vi "Teleop.vi"(10 "Match Info":T1={"Autonomous Elapsed Seconds"=0.0, "TeleOp Elapsed Seconds"=0.0, "Disabled Elapsed Seconds"=0.0, "Visited Autonomous"=FALSE, "Visited TeleOp"=FALSE, "Visited Disabled"=FALSE, "Autonomous Settings"={"Autonomous Style"=enum."Independent", "VI Refnum"=refnum}}, 11 "Call Context":T2) -> ()   [LabVIEW 2016]
doc: "This VI is called for each TeleOp packet received from the DS where the robot is not disabled. It is often used to read from the joysticks and update I/O or to update setpoints for timed control loops. It should complete and return within 20 milliseconds or it may miss DS packets."
uses:
  <vilib>/Rock Robotics/WPI/DriverStation/WPI_DriverStationDerivedRobotMode.ctl
  <vilib>/Rock Robotics/WPI/DriverStation/WPI_DriverStationMatch Info.ctl
  <vilib>/Rock Robotics/WPI/Relay/WPI_RelayValue.ctl
  <vilib>/Rock Robotics/WPI/Solenoid/WPI_SolenoidValue.ctl
  <vilib>/Rock Robotics/WPI/Utilities/WPI_GetSetVariantRefNum.vi
  <vilib>/Rock Robotics/Network Tables/NT Write Boolean Array.vi
  <vilib>/Rock Robotics/Network Tables/NT Write Numeric Array.vi
  <vilib>/Rock Robotics/Network Tables/NT Read Boolean.vi
  <vilib>/Rock Robotics/Network Tables/NT Read Number.vi
  <vilib>/Rock Robotics/WPI/Solenoid/WPI_SolenoidSetEnum.vi
panel:
  out "Feed 2":dbl(slide) scale=-1.0..1.0
  out "Feed":dbl(slide) scale=-1.0..1.0
  out "Sample Slider 0":dbl(slide) scale=0.0..5.0
  out "Sample Boolean 1":bool
  out "Sample Boolean 0":bool
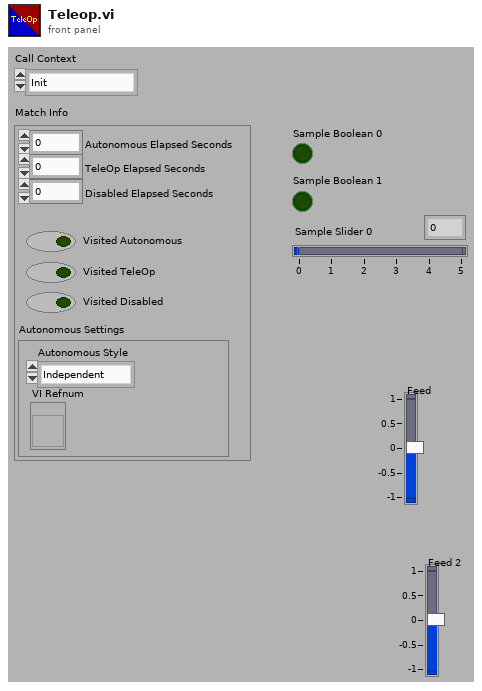
[diagram p1: front panel]
types:
  T1 = typedef "WPI_DriverStationMatch Info.ctl" = cluster{"Autonomous Elapsed Seconds":dbl, "TeleOp Elapsed Seconds":dbl, "Disabled Elapsed Seconds":dbl, "Visited Autonomous":bool, "Visited TeleOp":bool, "Visited Disabled":bool, "Autonomous Settings":cluster{"Autonomous Style":enum16{"Iterative", "Independent"}, "VI Refnum":refnum<vi>}}
  T2 = typedef "WPI_DriverStationDerivedRobotMode.ctl" = enum16{"Init", "Execute", "Stop"}
  T3 = typedef "WPI_JoystickDevRef.ctl" = cluster{"Device":T4}
  T4 = typedef "WPI_JoystickDeviceEnum.ctl" = enum16{"USB 0", "USB 1", "USB 2", "USB 3", "USB 4", "USB 5"}
  T5 = cluster{"Buttons[0]":bool, "Buttons[1]":bool, "Buttons[2]":bool, "Buttons[3]":bool, "Buttons[4]":bool, "Buttons[5]":bool, "Buttons[6]":bool, "Buttons[7]":bool, "Buttons[8]":bool, "Buttons[9]":bool, "Buttons[10]":bool}
  T6 = typedef "WPI_MotorControlDeviceRef.ctl" = cluster{"DeviceStatus":errorcluster, "Type":T7, "PWM":cluster{"PWM Channel":T8, "DeadBand":T9}, "CAN":cluster{"Device Number":u8, "SetOutput VI Ref":variant, "GetOutput VI Ref":variant, "Enable VI Ref":variant, "Disable VI Ref":variant, "Data":variant}, "Invert":bool}
  T7 = typedef "WPI_MotorControlType.ctl" = enum16{"PWM", "CAN"}
  T8 = typedef "FPGA_DIOPWMChannel.ctl" = enum8{"PWM 0", "PWM 1", "PWM 2", "PWM 3", "PWM 4", "PWM 5", "PWM 6", "PWM 7", "PWM 8", "PWM 9", "PWM MXP 0", "PWM MXP 1", "PWM MXP 2", "PWM MXP 3", "PWM MXP 4", "PWM MXP 5", "PWM MXP 6", "PWM MXP 7", "PWM MXP 8", "PWM MXP 9", "Invalid"}
  T9 = typedef "WPI_PWMDeadband.ctl" = cluster{"Name":string, "maxPositivePwm":i32, "minPositivePwm":i32, "centerPwm":i32, "maxNegativePwm":i32, "minNegativePwm":i32, "angularRange":u16}
  T10 = typedef "WPI_RelayDevRef.ctl" = cluster{"DevStatus":errorcluster, "Relay Channel":T11, "Relay Direction":T12}
  T11 = typedef "FPGA_DIORelayChannel.ctl" = enum8{"Relay 0", "Relay 1", "Relay 2", "Relay 3", "Invalid"}
  T12 = typedef "WPI_RelayDirection.ctl" = enum16{"Both directions", "Forward only", "Reverse only"}
  T13 = typedef "WPI_RobotDriveDevRef.ctl" = cluster{"DevStatus":errorcluster, "Motors[]":T6[], "Square Inputs":bool, "Max Output":dbl}
  T14 = typedef "WPI_SolenoidDevRef.ctl" = cluster{"DevStatus":errorcluster, "Pneumatics Control Module":u8, "Forward Solenoid Channel":T15, "Reverse Solenoid Channel":T15}
  T15 = typedef "WPI_SolenoidChannel.ctl" = enum8{"Solenoid 0", "Solenoid 1", "Solenoid 2", "Solenoid 3", "Solenoid 4", "Solenoid 5", "Solenoid 6", "Solenoid 7", "Invalid"}
  T16 = cluster{"Axes[0]":dbl, "Axes[1]":dbl, "Axes[2]":dbl, "Axes[3]":dbl, "Axes[4]":dbl, "Axes[5]":dbl, "Axes[6]":dbl, "Axes[7]":dbl, "Axes[8]":dbl}
  T17 = typedef "WPI_SolenoidValue.ctl" = enum16{"Off", "On", "Forward", "Reverse"}
  T18 = typedef "WPI_RelayValue.ctl" = enum16{"Off", "On", "Forward", "Reverse"}
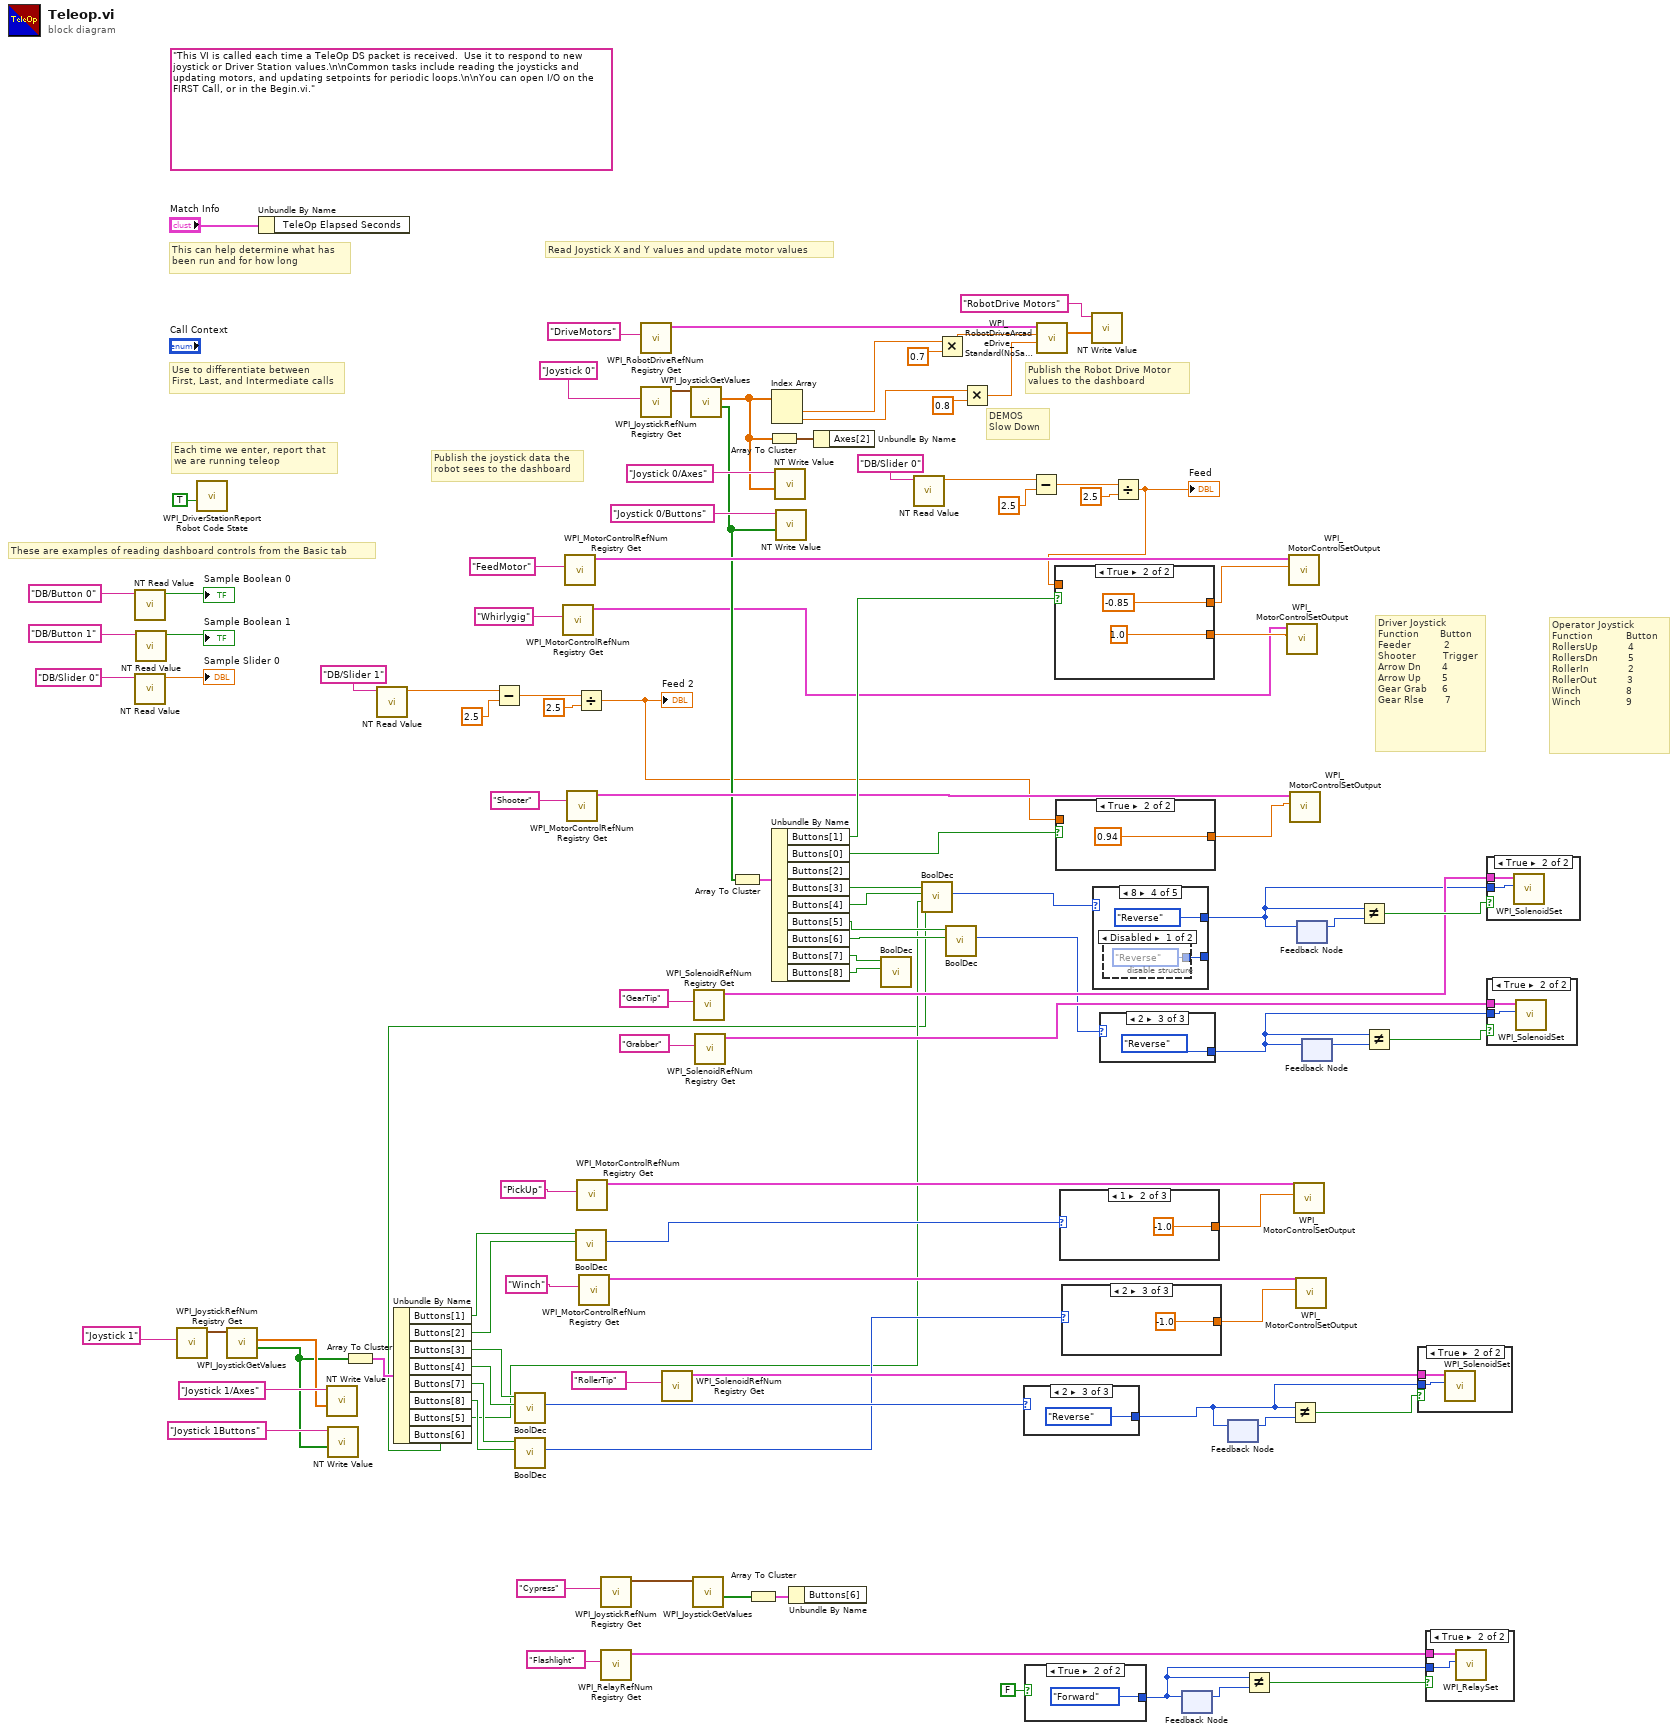
[diagram p0: block diagram]
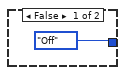
[diagram p3: hidden frame]
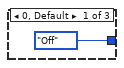
[diagram p4: hidden frame]
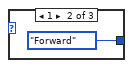
[diagram p5: hidden frame]
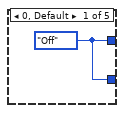
[diagram p6: hidden frame]
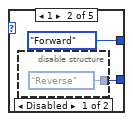
[diagram p7: hidden frame]
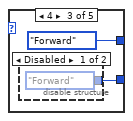
[diagram p9: hidden frame]
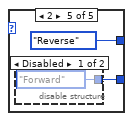
[diagram p12: hidden frame]
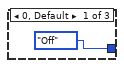
[diagram p17: hidden frame]
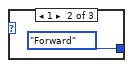
[diagram p18: hidden frame]
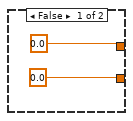
[diagram p19: hidden frame]
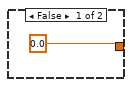
[diagram p20: hidden frame]
diagram:
  (unwired) "This VI is called each time a TeleOp DS packet is received.  Use it to respond to new joystick or Driver Station values.\n\nCommon tasks include reading the joysticks and updating motors, and updating setpoints for periodic loops.\n\nYou can open I/O on the FIRST Call, or in the Begin.vi."
  # "DEMOS\nSlow Down"
  # "Operator Joystick\nFunction           Button\nRollersUp          4\nRollersDn          5\nRollerIn             2\nRollerOut          3\nWinch               8\nWinch               9"
  # "Driver Joystick\nFunction       Button\nFeeder           2\nShooter         Trigger\nArrow Dn       4\nArrow Up       5\nGear Grab     6\nGear Rlse       7"
  # "These are examples of reading dashboard controls from the Basic tab"
  # "Publish the Robot Drive Motor\nvalues to the dashboard"
  # "Publish the joystick data the\nrobot sees to the dashboard"
  # "Each time we enter, report that\nwe are running teleop"
  # "Use to differentiate between\nFirst, Last, and Intermediate calls"
  # "This can help determine what has\nbeen run and for how long"
  # "Read Joystick X and Y values and update motor values"
  n1 = call-poly <vilib>:"NT Read Value.vi"("Name"="DB/Button 0" ("refnum name")) -> ("Boolean"=→"Sample Boolean 0":bool)  [unwired: 9 in, 1 out]
  n2 = call-poly <vilib>:"NT Read Value.vi"("Name"="DB/Slider 0" ("refnum name")) -> ("Numeric"=→"Sample Slider 0":dbl)  [unwired: 9 in, 1 out]
  n3 = call-poly <vilib>:"NT Read Value.vi"("Name"="DB/Button 1" ("refnum name")) -> ("Boolean"=→"Sample Boolean 1":bool)  [unwired: 9 in, 1 out]
  n4 = call <vilib>:"WPI_JoystickRefNum Registry Get.vi"("refnum name"="Joystick 1") -> ("JoystickDevRef"=w73:T3)  [unwired: 1 in, 9 out]
  n5 = call <vilib>:"WPI_DriverStationReport Robot Code State.vi"("TeleOp"=TRUE ("Autonomous")) -> ()  [unwired: 10 in, 1 out]
  n6 = call <vilib>:"WPI_JoystickGetValues.vi"("JoystickDevRef"=w73) -> ("Buttons"=w63:bool[], "Axes"=w69:dbl[])  [unwired: 6 in, 3 out]
  n7 = Unbundle By Name("Match Info") -> ()  [unwired: 1 out]
  n8 = call-poly <vilib>:"NT Write Value.vi"("Numeric Array"=w69, "Name"="Joystick 1/Axes") -> ()  [unwired: 9 in, 1 out]
  n9 = call-poly <vilib>:"NT Write Value.vi"("Boolean Array"=w63, "Name"="Joystick 1Buttons") -> ()  [unwired: 9 in, 1 out]
  n10 = Array To Cluster(array=w63) -> (cluster=w62:T5)
  n11 = call-poly <vilib>:"NT Read Value.vi"("Name"="DB/Slider 1") -> ("Numeric"=w37:dbl)  [unwired: 9 in, 1 out]
  n12 = Unbundle By Name(w62) -> ("Buttons[1]"=w59:bool, "Buttons[2]"=w58:bool, "Buttons[3]"=w61:bool, "Buttons[4]"=w60:bool, "Buttons[7]"=w53:bool, "Buttons[8]"=w52:bool, "Buttons[5]"=w8:bool, "Buttons[6]"=w7:bool)
  n13 = Subtract(x=w37, y=2.5) -> (x-y=w35:dbl)
  n14 = call "BoolDec.vi"("Bit0"=w61, "Bit1"=w60) -> ("Out"=w22:i8)  [unwired: 8 in]
  n15 = call "BoolDec.vi"("Bit0"=w53, "Bit1"=w52) -> ("Out"=w20:i8)  [unwired: 8 in]
  n16 = call <vilib>:"WPI_MotorControlRefNum Registry Get.vi"("refnum name"="Whirlygig") -> ("MotorControlDevRef"=w4:T6)  [unwired: 9 in, 1 out]
  n17 = call <vilib>:"WPI_MotorControlRefNum Registry Get.vi"("refnum name"="FeedMotor") -> ("MotorControlDevRef"=w76:T6)  [unwired: 9 in, 1 out]
  n18 = call <vilib>:"WPI_MotorControlRefNum Registry Get.vi"("refnum name"="Shooter") -> ("MotorControlDevRef"=w77:T6)  [unwired: 9 in, 1 out]
  n19 = Divide(x=w35, y=2.5) -> (x/y=w27:dbl)
  "Feed 2" <- w27
  n20 = call "BoolDec.vi"("Bit0"=w59, "Bit1"=w58) -> ("Out"=w21:i8)  [unwired: 8 in]
  n21 = call <vilib>:"WPI_MotorControlRefNum Registry Get.vi"("refnum name"="PickUp") -> ("MotorControlDevRef"=w86:T6)  [unwired: 9 in, 1 out]
  n22 = call <vilib>:"WPI_MotorControlRefNum Registry Get.vi"("refnum name"="Winch") -> ("MotorControlDevRef"=w81:T6)  [unwired: 9 in, 1 out]
  n23 = call <vilib>:"WPI_JoystickRefNum Registry Get.vi"("refnum name"="Cypress") -> ("JoystickDevRef"=w18:T3)  [unwired: 9 in, 1 out]
  n24 = call <vilib>:"WPI_RelayRefNum Registry Get.vi"("refnum name"="Flashlight") -> ("RelayDevRef"=w32:T10)  [unwired: 9 in, 1 out]
  n25 = call <vilib>:"WPI_RobotDriveRefNum Registry Get.vi"("refnum name"="DriveMotors") -> ("RobotDriveDevRef"=w104:T13)  [unwired: 1 in, 9 out]
  n26 = call <vilib>:"WPI_JoystickRefNum Registry Get.vi"("refnum name"="Joystick 0") -> ("JoystickDevRef"=w102:T3)  [unwired: 1 in, 9 out]
  n27 = call <vilib>:"WPI_SolenoidRefNum Registry Get.vi"("refnum name"="RollerTip") -> ("SolenoidDevRef"=w64:T14)  [unwired: 9 in, 1 out]
  n28 = call <vilib>:"WPI_JoystickGetValues.vi"("JoystickDevRef"=w102) -> ("Buttons"=w68:bool[], "Axes"=w88:dbl[])  [unwired: 6 in, 3 out]
  n29 = call <vilib>:"WPI_JoystickGetValues.vi"("JoystickDevRef"=w18) -> ("Buttons"=w17:bool[])  [unwired: 6 in, 4 out]
  n30 = call <vilib>:"WPI_SolenoidRefNum Registry Get.vi"("refnum name"="GearTip") -> ("SolenoidDevRef"=w25:T14)  [unwired: 9 in, 1 out]
  n31 = call <vilib>:"WPI_SolenoidRefNum Registry Get.vi"("refnum name"="Grabber") -> ("SolenoidDevRef"=w24:T14)  [unwired: 9 in, 1 out]
  n32 = Array To Cluster(array=w68) -> (cluster=w89:T5)
  n33 = Array To Cluster(array=w17) -> (cluster=w16:T5)
  n34 = Array To Cluster(array=w88) -> (cluster=w87:T16)
  n35 = Index Array(array=w88) -> (element #1=w46:dbl, element #2=w2:dbl)  [unwired: 2 in]
  n36 = Unbundle By Name(w89) -> ("Buttons[1]"=w78:bool, "Buttons[0]"=w79:bool, "Buttons[3]"=w9:bool, "Buttons[4]"=w26:bool, "Buttons[5]"=w15:bool, "Buttons[6]"=w14:bool, "Buttons[7]"=w84:bool, "Buttons[8]"=w83:bool)  [unwired: 1 out]
  n37 = call-poly <vilib>:"NT Write Value.vi"("Numeric Array"=w88, "Name"="Joystick 0/Axes") -> ()  [unwired: 9 in, 1 out]
  n38 = call-poly <vilib>:"NT Write Value.vi"("Boolean Array"=w68, "Name"="Joystick 0/Buttons") -> ()  [unwired: 9 in, 1 out]
  n39 = Unbundle By Name(w16) -> ()  [unwired: 1 out]
  n40 = Unbundle By Name(w87) -> ()  [unwired: 1 out]
  n41 = call "BoolDec.vi"("Bit0"=w84, "Bit1"=w83) -> ()  [unwired: 8 in, 1 out]
  n42 = call-poly <vilib>:"NT Read Value.vi"("Name"="DB/Slider 0") -> ("Numeric"=w43:dbl)  [unwired: 9 in, 1 out]
  n43 = call "BoolDec.vi"("Bit0"=w9, "Bit1"=w26, "Bit2"=w8, "Bit3"=w7) -> ("Out"=w13:i8)  [unwired: 6 in]
  n44 = Multiply(x=w46, y=0.7) -> (x*y=w10:dbl)
  n45 = call "BoolDec.vi"("Bit0"=w15, "Bit1"=w14) -> ("Out"=w23:i8)  [unwired: 8 in]
  n46 = Multiply(x=w2, y=0.8) -> (x*y=w1:dbl)
  n47 = case shown="2" w22 {
    tunnel: [WPI_SolenoidValue."Off" ("Value") WPI_SolenoidValue."Forward" ("Value") WPI_SolenoidValue."Reverse" ("Value")] -> w49
    frame 0, Default {
    }
    frame 1 {
    }
    frame 2 {
    }
  }
  n48 = case shown="True" FALSE {
    tunnel: [WPI_RelayValue."Off" ("RelayValue") WPI_RelayValue."Forward" ("RelayValue")] -> w28
    frame False {
    }
    frame True {
    }
  }
  n49 = Subtract(x=w43, y=2.5) -> (x-y=w41:dbl)
  n50 = call <vilib>:"WPI_RobotDriveArcadeDrive_Standard(NoSaturation).vi"("Y axis value"=w1, "X axis value"=w10, "RobotDriveDevRef"=w104) -> ("Motor Values"=w92:dbl[])  [unwired: 1 in, 7 out]
  n51 = case shown="True" w79 {
    tunnel: [0.0 ("Output") 0.94] -> w47
    tunnel: w27 -> [_ _]
    frame False {
    }
    frame True {
    }
  }
  n52 = case shown="1" w21 {
    tunnel: [0.0 ("Output") -1.0 1.0] -> w85
    frame 0, Default {
    }
    frame 1 {
    }
    frame 2 {
    }
  }
  n53 = case shown="2" w20 {
    tunnel: [0.0 ("Output") 1.0 -1.0] -> w82
    frame 0, Default {
    }
    frame 1 {
    }
    frame 2 {
    }
  }
  n54 = call-poly <vilib>:"NT Write Value.vi"("Numeric Array"=w92, "Name"="RobotDrive Motors") -> ()  [unwired: 9 in, 1 out]
  n55 = case shown="8" w13 {
    tunnel: [w120 WPI_SolenoidValue."Forward" ("Value") WPI_SolenoidValue."Forward" ("Value") WPI_SolenoidValue."Reverse" ("Value") WPI_SolenoidValue."Reverse" ("Value")] -> w12
    tunnel: [w120 w121 w124 w127 w130] -> _
    frame 0, Default {
      w120 = WPI_SolenoidValue."Off" ("Value")
    }
    frame 1 {
      n56 = disable-structure shown="Disabled" {
        disable-tunnel: [WPI_SolenoidValue."Reverse" ("Value") _] -> w121
        frame Disabled {
        }
        frame Enabled {
        }
      }
    }
    frame 4 {
      n57 = disable-structure shown="Disabled" {
        disable-tunnel: [WPI_SolenoidValue."Forward" ("Value") _] -> w124
        frame Disabled {
        }
        frame Enabled {
        }
      }
    }
    frame 8 {
      n58 = disable-structure shown="Disabled" {
        disable-tunnel: [WPI_SolenoidValue."Reverse" ("Value") _] -> w127
        frame Disabled {
        }
        frame Enabled {
        }
      }
    }
    frame 2 {
      n59 = disable-structure shown="Disabled" {
        disable-tunnel: [WPI_SolenoidValue."Forward" ("Value") _] -> w130
        frame Disabled {
        }
        frame Enabled {
        }
      }
    }
  }
  n60 = case shown="2" w23 {
    tunnel: [WPI_SolenoidValue."Off" ("Value") WPI_SolenoidValue."Forward" ("Value") WPI_SolenoidValue."Reverse" ("Value")] -> w11
    frame 0, Default {
    }
    frame 1 {
    }
    frame 2 {
    }
  }
  n61 = Divide(x=w41, y=2.5) -> (x/y=w39:dbl)
  "Feed" <- w39
  n62 = case shown="True" w78 {
    tunnel: [0.0 ("Output") -0.85] -> w48
    tunnel: w39 -> [_ _]
    tunnel: [0.0 ("Output") 1.0] -> w5
    frame False {
    }
    frame True {
    }
  }
  n63 = feedback #1() -> (w31:T18)  [unwired: 1 in]
  n64 = feedback-in #1(w28) -> ()
  n65 = feedback #2() -> (w54:T17)  [unwired: 1 in]
  n66 = feedback-in #2(w49) -> ()
  n67 = Not Equal?(x=w28, y=w31) -> (x != y?=w30:bool)
  n68 = call <vilib>:"WPI_MotorControlSetOutput.vi"("Output"=w5, "MotorControlDevRef"=w4) -> ()  [unwired: 7 in, 3 out]
  n69 = call <vilib>:"WPI_MotorControlSetOutput.vi"("Output"=w48, "MotorControlDevRef"=w76) -> ()  [unwired: 7 in, 3 out]
  n70 = call <vilib>:"WPI_MotorControlSetOutput.vi"("Output"=w47, "MotorControlDevRef"=w77) -> ()  [unwired: 7 in, 3 out]
  n71 = Not Equal?(x=w49, y=w54) -> (x != y?=w50:bool)
  n72 = call <vilib>:"WPI_MotorControlSetOutput.vi"("Output"=w85, "MotorControlDevRef"=w86) -> ()  [unwired: 7 in, 3 out]
  n73 = call <vilib>:"WPI_MotorControlSetOutput.vi"("Output"=w82, "MotorControlDevRef"=w81) -> ()  [unwired: 7 in, 3 out]
  n74 = feedback #3() -> (w55:T17)  [unwired: 1 in]
  n75 = feedback-in #3(w12) -> ()
  n76 = feedback-in #4(w11) -> ()
  n77 = feedback #4() -> (w56:T17)  [unwired: 1 in]
  n78 = Not Equal?(x=w12, y=w55) -> (x != y?=w51:bool)
  n79 = Not Equal?(x=w11, y=w56) -> (x != y?=w57:bool)
  n80 = case shown="True" w50 {
    tunnel: w64 -> [_ w141]
    tunnel: w49 -> [_ w140]
    frame False {
    }
    frame True {
      n81 = call-poly <vilib>:"WPI_SolenoidSet.vi"("Value"=w140, "SolenoidDevRef"=w141) -> ()  [unwired: 8 in, 2 out]
    }
  }
  n82 = case shown="True" w30 {
    tunnel: w32 -> [_ w143]
    tunnel: w28 -> [_ w142]
    frame False {
    }
    frame True {
      n83 = call <vilib>:"WPI_RelaySet.vi"("RelayValue"=w142, "RelayDevRef"=w143) -> ()  [unwired: 8 in, 2 out]
    }
  }
  n84 = case shown="True" w51 {
    tunnel: w25 -> [_ w145]
    tunnel: w12 -> [_ w144]
    frame False {
    }
    frame True {
      n85 = call-poly <vilib>:"WPI_SolenoidSet.vi"("Value"=w144, "SolenoidDevRef"=w145) -> ()  [unwired: 8 in, 2 out]
    }
  }
  n86 = case shown="True" w57 {
    tunnel: w24 -> [_ w147]
    tunnel: w11 -> [_ w146]
    frame False {
    }
    frame True {
      n87 = call-poly <vilib>:"WPI_SolenoidSet.vi"("Value"=w146, "SolenoidDevRef"=w147) -> ()  [unwired: 8 in, 2 out]
    }
  }
